vi "Load SequenceFile.vi"(8 "error in (no error)":errorcluster, 10 "SequenceFile":refnum<class "SequenceFile.lvclass">, 11 "SequenceViewPanel in":refnum<class "SequenceViewPanel.lvclass">) -> (0 "error out":errorcluster, 3 "SequenceViewPanel out":refnum<class "SequenceViewPanel.lvclass">)   [LabVIEW 2020, in "TSnax UI.lvlib" / "SequenceViewPanel.lvclass"]
uses:
  SequenceViewPanel.lvclass
  TSnax/SequenceFile/SequenceFile.lvclass
  SequenceViewPanel.lvclass/SequenceViewPanel.ctl
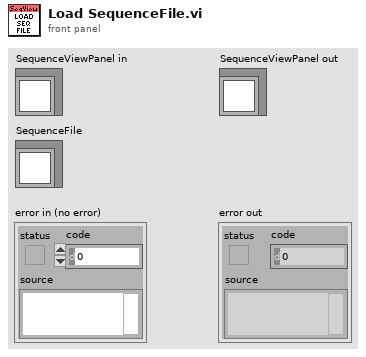
[diagram p1: front panel]
types:
  T1 = typedef "TSnax UI.lvlib/SequenceViewPanel.lvclass/Ref Data.ctl" = cluster{"Insert Index":i32, "SequenceFile":refnum<class "SequenceFile.lvclass">}
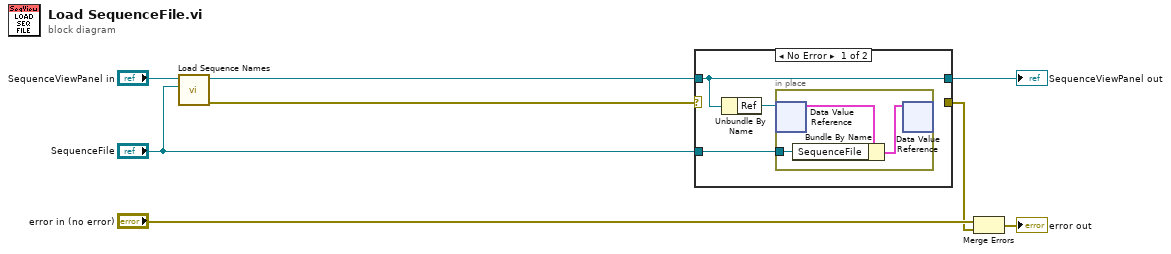
[diagram p0: block diagram]
diagram:
  n1 = call "Load Sequence Names.vi"("SequenceFile"="SequenceFile", "SequenceViewPanel in"="SequenceViewPanel in") -> ("error out"=w5:errorcluster, "SequenceViewPanel out"=w6:refnum<class "SequenceViewPanel.lvclass">)  [unwired: 8 in]
  n2 = case shown="No Error" w5 {
    selector: w5 -> [_ w16]
    tunnel: w6 -> [w9 w15]
    tunnel: "SequenceFile" -> [w10 _]
    tunnel: [w9 w15] -> w3
    tunnel: [_ w16] -> w1
    frame No Error {
      n3 = Unbundle By Name(w9) -> ("Ref"=w11:refnum<data-value>)
      n4 = in-place {
        in-place-border: w10 -> [w12]
        n5 = in-place-dvr #1(w11) -> (w14:T1)  [unwired: 1 out]
        n6 = Bundle By Name(cluster=w14, "SequenceFile"=w12) -> (w13:T1)
        n7 = in-place-dvr #1(w13) -> ()  [unwired: 2 out]
      }
    }
    frame Error {
    }
  }
  "SequenceViewPanel out" <- w3
  n8 = Merge Errors("error in (no error)", w1) -> (→"error out":errorcluster)
